vi "Sequence (Express).vi"() -> ()   [LabVIEW 2011]
doc: "The Sequence (Express) VI acquires a sequence of images and displays the images in an image control usingthe Vision Acquisition Express VI. A sequence is appropriate for applications in which you want to process multiple images."
uses:
  Instance           1 26Saved   Sequence (Express) .vi
panel:
  in  "Stop":bool
  out "Image Array":T1[](array[plugin-control])
  in  "Number of Images":u32=5
  # "Overview: Demonstrates how to acquire a sequence of images and displays them in an array of image display controls..\nRequirements: Vision Acquisition Software\nInstructions: Run the VI"
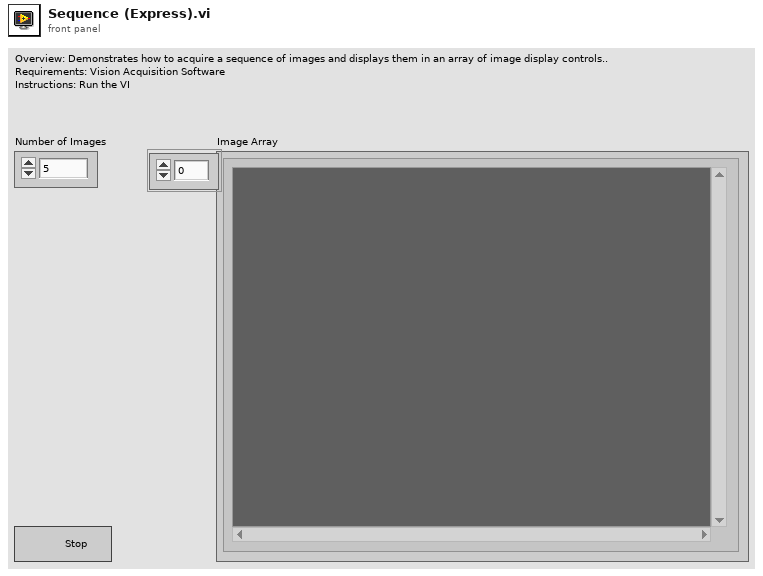
[diagram p1: front panel]
types:
  T1 = typedef "IMAQ Image.ctl" = refnum<image>
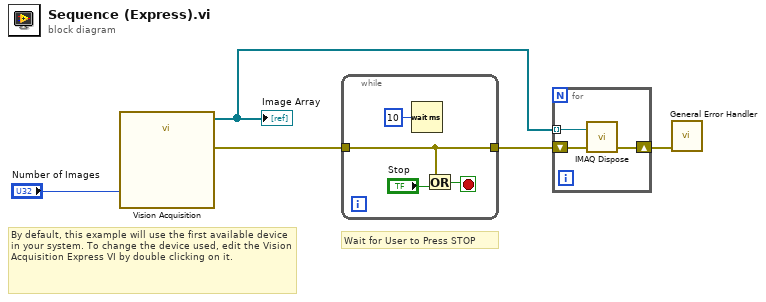
[diagram p0: block diagram]
diagram:
  # "Wait for User to Press STOP"
  # "By default, this example will use the first available device in your system. To change the device used, edit the Vision Acquisition Express VI by double clicking on it."
  n1 = call "Vision Acquisition"("Number of Images"="Number of Images") -> ("All Images Out"=w1:T1[], "error out"=w3:errorcluster)  [unwired: 1 in, 24 out]
  "Image Array" <- w1
  n2 = while {
    tunnel: [w6] -> w4
    tunnel: w3 -> [w6]
    stop <- w7 stop-if-true
    n3 = Wait (ms)(milliseconds to wait=u32 10) -> ()  [unwired: 1 out]
    n4 = Or(x=w6, y="Stop") -> (x .or. y?=w7:bool)
  }
  n5 = for {
    tunnel: w1 -> [w12] mode=indexing
    shift-right: [w10] -> w2
    shift-left: w4 -> [w11]
    n6 = call "IMAQ Dispose"("Image"=w12, "error in (no error)"=w11) -> ("error out"=w10:errorcluster)  [unwired: 1 in, 3 out]
  }
  n7 = call <vilib>:"General Error Handler.vi"("error in (no error)"=w2) -> ()  [unwired: 1 in, 14 out]
